vi "Set Channel Data.vi"(6 "waveform":waveform(dbl), 7 "data type":T1, 8 "error in":errorcluster, 9 "double channel data":dbl[](array[numeric]), 10 "I16 channel data":i16[](array[numeric]), 11 "TDMS in":refnum<class "TDMS.lvclass">) -> (0 "error out":errorcluster, 3 "TDMS out":refnum<class "TDMS.lvclass">)   [LabVIEW 2011, in "TDMS.lvclass"]
uses:
  TDMS.lvclass
  Data Type.ctl
  TDMS.lvclass/TDMS.ctl
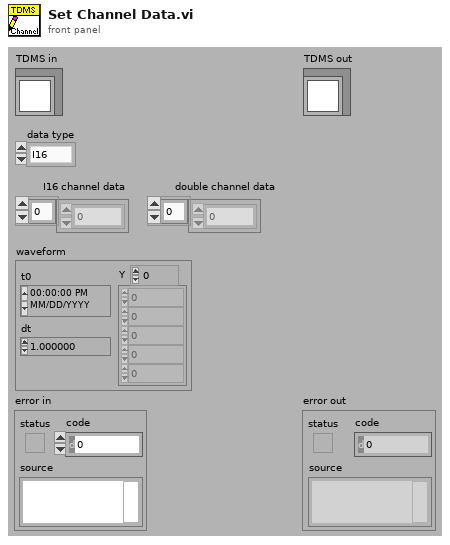
[diagram p1: front panel]
types:
  T1 = typedef "TDMS.lvclass/Data Type.ctl" = enum16{"I16", "Double", "Waveform"}
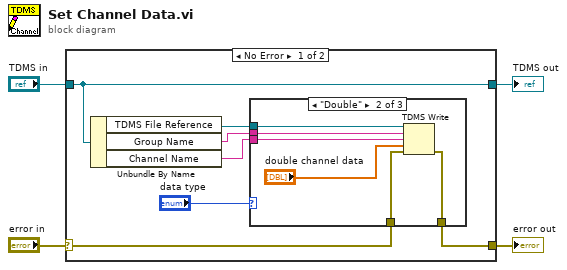
[diagram p0: block diagram]
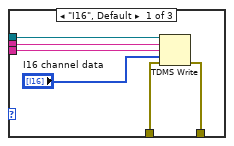
[diagram p2: hidden frame]
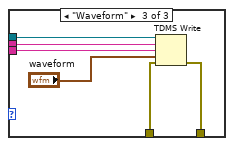
[diagram p3: hidden frame]
diagram:
  n1 = case shown="No Error" "error in" {
    selector: "error in" -> [w6 w31]
    tunnel: [w5 w31] -> w3
    tunnel: "TDMS in" -> [w11 w30]
    tunnel: [w11 w30] -> w1
    frame No Error {
      n2 = Unbundle By Name(w11) -> ("TDMS File Reference"=w10:refnum<k34>, "Group Name"=w9:string, "Channel Name"=w8:string)
      n3 = case shown="\"Double\"" "data type" {
        tunnel: w10 -> [w17 w23 w29]
        tunnel: w9 -> [w16 w22 w28]
        tunnel: w8 -> [w14 w21 w27]
        tunnel: w6 -> [w13 w19 w25]
        tunnel: [w12 w18 w24] -> w5
        frame "I16", Default {
          n4 = TDMS Write(0:w17, 5:w16, 7:w14, 9:"I16 channel data", 11:w13) -> (15:w12:errorcluster)  [unwired: 1 in, 3 out]
        }
        frame "Double" {
          n5 = TDMS Write(0:w23, 5:w22, 7:w21, 9:"double channel data", 11:w19) -> (15:w18:errorcluster)  [unwired: 1 in, 3 out]
        }
        frame "Waveform" {
          n6 = TDMS Write(0:w29, 5:w28, 7:w27, 9:"waveform", 11:w25) -> (15:w24:errorcluster)  [unwired: 1 in, 3 out]
        }
      }
    }
    frame Error {
    }
  }
  "error out" <- w3
  "TDMS out" <- w1
